vi "Missile Fire.vi"(9 "Right Stick in":cluster{dbl, dbl}, 11 "Flying Saucer in":refnum<class "Flying Saucer.lvclass">) -> (2 "Missile out":refnum<class "Missile.lvclass">, 3 "Flying Saucer out":refnum<class "Flying Saucer.lvclass">)   [LabVIEW 2024, in "Flying Saucer.lvclass"]
doc: "MIT Licence\nCopyright (c) 2024 David Grollier"
uses:
  Flying Saucer.lvclass
  Missile/Missile.lvclass
  Game Componants.lvclass/Game Componants.ctl
  Movable.lvclass/Movable.ctl
  <vilib>/Analysis/_algsub.llb/Vector Norm.vi
  <vilib>/Analysis/_algsub.llb/Real Vector Norm.vi
  Game Board/Game Board.lvclass
  Movable.lvclass
  Game Componants.lvclass
  Utils/Utils.lvlib
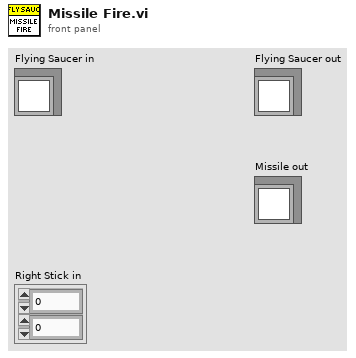
[diagram p1: front panel]
types:
  T1 = typedef "Coordinates.ctl" = cluster{"x":dbl, "y":dbl}
  T2 = typedef "Velocity.ctl" = cluster{"Vx":dbl, "Vy":dbl}
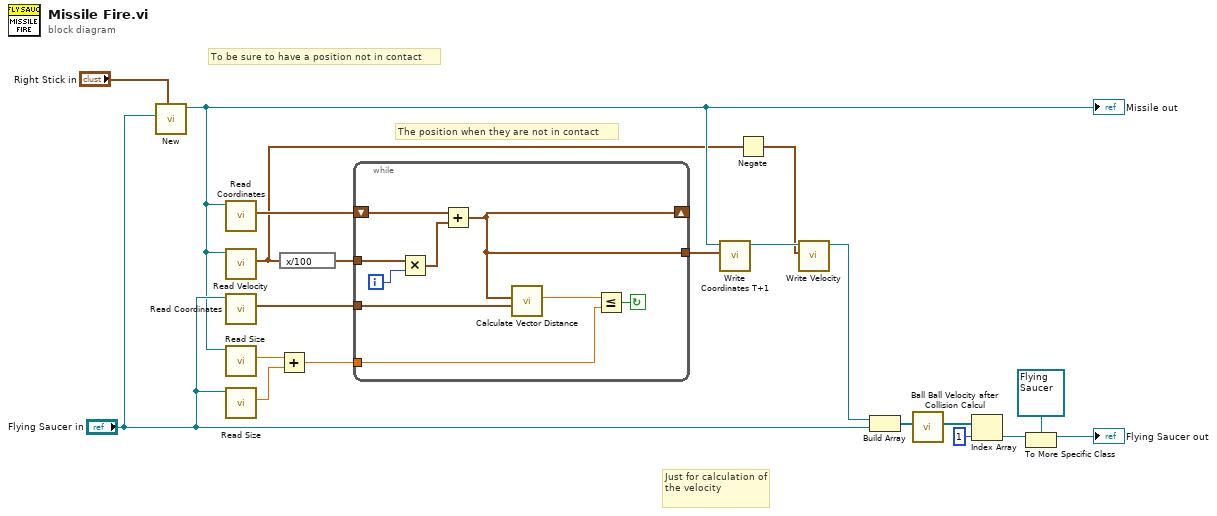
[diagram p0: block diagram]
diagram:
  # "To be sure to have a position not in contact"
  # "Just for calculation of the velocity"
  # "The position when they are not in contact"
  n1 = call "New.vi"("Velocity direction in"="Right Stick in", "Flying saucer in"="Flying Saucer in") -> ("Missile out"=w6:refnum<class "Missile.lvclass">)  [unwired: 9 in]
  "Missile out" <- w6
  n2 = call "Read Coordinates.vi"("Game Componants in"=w6) -> ("Coordinates"=w7:T1)  [unwired: 10 in]
  n3 = call-dynamic "Read Velocity.vi"("Movable in"=w6) -> ("Velocity"=w2:T2)  [unwired: 10 in]
  n4 = call "Read Coordinates.vi"("Game Componants in"="Flying Saucer in") -> ("Coordinates"=w11:T1)  [unwired: 10 in]
  n5 = call "Read Size.vi"("Movable in"=w6) -> ("Size"=w18:dbl)  [unwired: 10 in]
  n6 = call "Read Size.vi"("Movable in"="Flying Saucer in") -> ("Size"=w17:dbl)  [unwired: 10 in]
  n7 = Add(x=w18, y=w17) -> (x+y=w19:dbl)
  n8 = expression code="x/100"(w2) -> (w5:T2)
  n9 = while {
    tunnel: w19 -> [w29]
    tunnel: w11 -> [w22]
    tunnel: [w23] -> w16
    shift-right: [w23] -> _
    shift-left: w7 -> [w27]
    tunnel: w5 -> [w26]
    i -> [w25]
    stop <- w28 continue-if-true
    n10 = Multiply(x=w26, y=w25) -> (x*y=w24:T2)
    n11 = Add(x=w27, y=w24) -> (x+y=w23:T1)
    n12 = call "Calculate Vector Distance.vi"("V2"=w22, "V1"=w23) -> ("Distance out"=w21:dbl)  [unwired: 9 in]
    n13 = Less Or Equal?(x=w21, y=w29) -> (x <= y?=w28:bool)
  }
  n14 = call "Write Coordinates T+1.vi"("Coordinates"=w16, "Movable in"=w6) -> ("Movable out"=w12:refnum<class "Missile.lvclass">)  [unwired: 9 in]
  n15 = Negate(x=w2) -> (-x=w1:T2)
  n16 = call "Write Velocity.vi"("Velocity"=w1, "Movable in"=w12) -> ("Movable out"=w3:refnum<class "Missile.lvclass">)  [unwired: 9 in]
  n17 = Build Array(w3, "Flying Saucer in") -> (w15:refnum<class "Movable.lvclass">[])
  n18 = call "Ball Ball Velocity after Collision Calcul.vi"("Movables in"=w15) -> ("Movables out"=w20:refnum<class "Movable.lvclass">[])  [unwired: 10 in]
  n19 = Index Array(array=w20, index=1) -> (element=w10:refnum<class "Movable.lvclass">)
  n20 = To More Specific Class(target class=refnum<class "Flying Saucer.lvclass"> refnum, reference=w10) -> (specific class reference=→"Flying Saucer out":refnum<class "Flying Saucer.lvclass">)  [unwired: 1 in, 1 out]
